vi "Get Ingredients.vi"(8 "error in (no error)":errorcluster, 11 "Logic Circuit in":refnum<class "Logic Circuit.lvclass">) -> (0 "error out":errorcluster, 2 "Ingredients":T1[](array[typedef]), 3 "Logic Circuit out":refnum<class "Logic Circuit.lvclass">)   [LabVIEW 2020, in "Logic Circuit.lvclass"]
uses:
  Logic Circuit.lvclass
  Item/Ingredient.ctl
  Item/Item.lvclass
  Simple Circuit/Simple Circuit.lvclass
  C:/dev/LabVIEW/Good Company Calc/Item/Item.lvclass
  Electronic Parts/Electronic Parts.lvclass
  Plastic Parts/Plastic Parts.lvclass
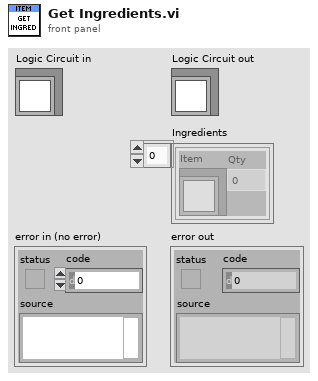
[diagram p1: front panel]
types:
  T1 = typedef "Item.lvclass/Ingredient.ctl" = cluster{"Item":refnum<class "Item.lvclass">, "Qty":dbl}
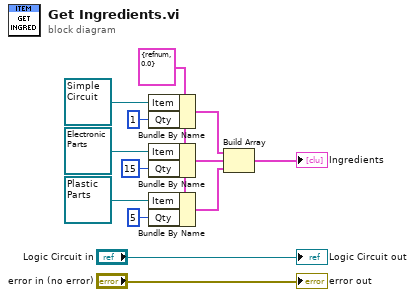
[diagram p0: block diagram]
diagram:
  w8 = T1 {"Item"=refnum, "Qty"=0.0} ("Ingredient")
  n1 = Bundle By Name(cluster=w8, "Item"=refnum<class "Simple Circuit.lvclass"> refnum ("Simple Circuit.lvclass"), "Qty"=1) -> (w5:T1)
  n2 = Bundle By Name(cluster=w8, "Item"=refnum<class "Electronic Parts.lvclass"> refnum ("Electronic Parts.lvclass"), "Qty"=15) -> (w7:T1)
  n3 = Bundle By Name(cluster=w8, "Item"=refnum<class "Plastic Parts.lvclass"> refnum ("Plastic Parts.lvclass"), "Qty"=5) -> (w6:T1)
  n4 = Build Array(w5, w7, w6) -> (→"Ingredients":T1[])
  "error out" <- "error in (no error)"
  "Logic Circuit out" <- "Logic Circuit in"
